vi "create single curve files.vi"(9 "Mea name":string, 10 "Sample Name":string, 11 "folder path":path) -> (1 "file name":string, 2 "xml path":path, 3 "data path":path)   [LabVIEW 2024]
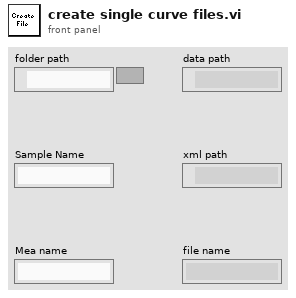
[diagram p1: front panel]
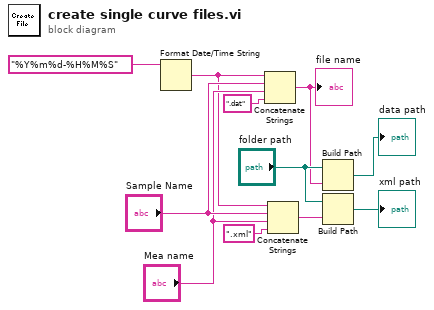
[diagram p0: block diagram]
diagram:
  n1 = Format Date/Time String(time format string (%c)="%Y%m%d-%H%M%S") -> (date/time string=w8:string)  [unwired: 2 in]
  n2 = Concatenate Strings(w8, "Sample Name", "Mea name", ".dat" ("string")) -> (w5:string)
  "file name" <- w5
  n3 = Concatenate Strings(w8, "Sample Name", "Mea name", ".xml" ("string")) -> (w2:string)
  n4 = Build Path(base path="folder path", name or relative path=w5) -> (appended path=→"data path":path)
  n5 = Build Path(base path="folder path", name or relative path=w2) -> (appended path=→"xml path":path)
